vi "Set_Control_Values.vi"(0 "Devices in":T18, 1 "Settings message":T1, 3 "Set Mode":T3, 4 "Timer parameters in":refnum<vi>, 5 "Main Parameters in":T4={"Mode"={"Mode"=enum."Dialog", "Expert?"=FALSE, "Dialog?"=FALSE}, "Stop loop"={"Settings changed?"=FALSE, "Stop?"=refnum}, "Send message"={"Send mode"=enum."Get parameters", "Set parameter list"=0, "Get parameter list"=0, "Reset device"=0, "Length set settings message"=0, "Reset buttons?"=FALSE, "Reset Master?"=enum."General"}, "Write settings"={"Options"=enum."File 1"}, "Settings state"={"MAS locked?"=refnum, "SLV locked?"=refnum}, "Button refs"={"Stop program"=refnum, "Save settings"=refnum, "DAQ mode"=refnum, "Reset settings"=refnum, "Apply settings"=refnum, "Reset MAS"=refnum, "Reset SLV"=refnum, "Local DBase?"=refnum, "Last value DBase"=FALSE, "Database"=refnum, "Calibration"=refnum, "Save settings 2"=refnum}, "Update screen"={"Detector number"=0, "Hardware"=enum."None"}, "Files"={"Path config file"=path "", "Path def. ini file"=path "", "Path ini file 1"=path "", "Path ini file 2"=path "", "Path RBF file"=path ""}, "DB connection"={"connection reference"=refnum, "Connected?"=refnum, "ODBC Name"=""}, "Status_id"=refnum, "Time difference"=refnum, "Satellites"=refnum, "Alignment parameters"=refnum, "Page Statistics 2"=refnum, "Database"=refnum, "Page Statistics"=refnum} {"Update screen"."Detector number" format="%#.0f"; "Send message"."Reset device" format="%x"; "Send message"."Get parameter list" format="%x"; "Send message"."Set parameter list" format="%x"}, 9 "Control Parameters [] in":T19[](array[typedef]) {"Aux Byte Value" format="%02x"; "Max Real Value" format="%#_6e"; "Min Real Value" format="%#_6e"; "dReal/dByte" format="%#_6e"; "Byte Value" format="%02x"; "Identifier" format="%02x"}, 11 "Status/Errors in":refnum<vi>) -> (6 "Main parameters out":T4={"Mode"={"Mode"=enum."Dialog", "Expert?"=FALSE, "Dialog?"=FALSE}, "Stop loop"={"Settings changed?"=FALSE, "Stop?"=refnum}, "Send message"={"Send mode"=enum."Get parameters", "Set parameter list"=0, "Get parameter list"=0, "Reset device"=0, "Length set settings message"=0, "Reset buttons?"=FALSE, "Reset Master?"=enum."General"}, "Write settings"={"Options"=enum."File 1"}, "Settings state"={"MAS locked?"=refnum, "SLV locked?"=refnum}, "Button refs"={"Stop program"=refnum, "Save settings"=refnum, "DAQ mode"=refnum, "Reset settings"=refnum, "Apply settings"=refnum, "Reset MAS"=refnum, "Reset SLV"=refnum, "Local DBase?"=refnum, "Last value DBase"=FALSE, "Database"=refnum, "Calibration"=refnum, "Save settings 2"=refnum}, "Update screen"={"Detector number"=0, "Hardware"=enum."None"}, "Files"={"Path config file"=path "", "Path def. ini file"=path "", "Path ini file 1"=path "", "Path ini file 2"=path "", "Path RBF file"=path ""}, "DB connection"={"connection reference"=refnum, "Connected?"=refnum, "ODBC Name"=""}, "Status_id"=refnum, "Time difference"=refnum, "Satellites"=refnum, "Alignment parameters"=refnum, "Page Statistics 2"=refnum, "Database"=refnum, "Page Statistics"=refnum} {"Update screen"."Detector number" format="%#.0f"; "Send message"."Reset device" format="%x"; "Send message"."Get parameter list" format="%x"; "Send message"."Set parameter list" format="%x"}, 8 "Run twice?":bool, 10 "Control Parameters [] out":T19[](array[typedef]) {"Aux Byte Value" format="%02x"; "Max Real Value" format="%#_6e"; "Min Real Value" format="%#_6e"; "dReal/dByte" format="%#_6e"; "Byte Value" format="%02x"; "Identifier" format="%02x"}, 12 "Slave Settings Message":T1, 14 "Master Settings Message":T1, 15 "Settings ok?":bool)   [LabVIEW 2013]
uses:
  Controls/Control_Parameters.ctl
  Controls/Master.ctl
  Controls/Devices.ctl
  Controls/Main_Parameters.ctl
  Controls/Mode.ctl
  Controls/Stop_Loop.ctl
  Controls/Send_Message.ctl
  Controls/Send_Message_Mode.ctl
  Controls/Write_Settings.ctl
  Controls/Write_Settings_Options.ctl
  Controls/Settings_State.ctl
  Controls/Button_Refs.ctl
  Controls/Update_Screen.ctl
  Controls/Files.ctl
  Controls/DB_Connection.ctl
  database/Connection.llb/Conn ObjectReference.ctl
  Controls/Settings_Message.ctl
  Controls/Setting.ctl
  Controls/Set_Mode.ctl
  Controls/Get_Set_Device_Options.ctl
  Controls/Device_Elements.ctl
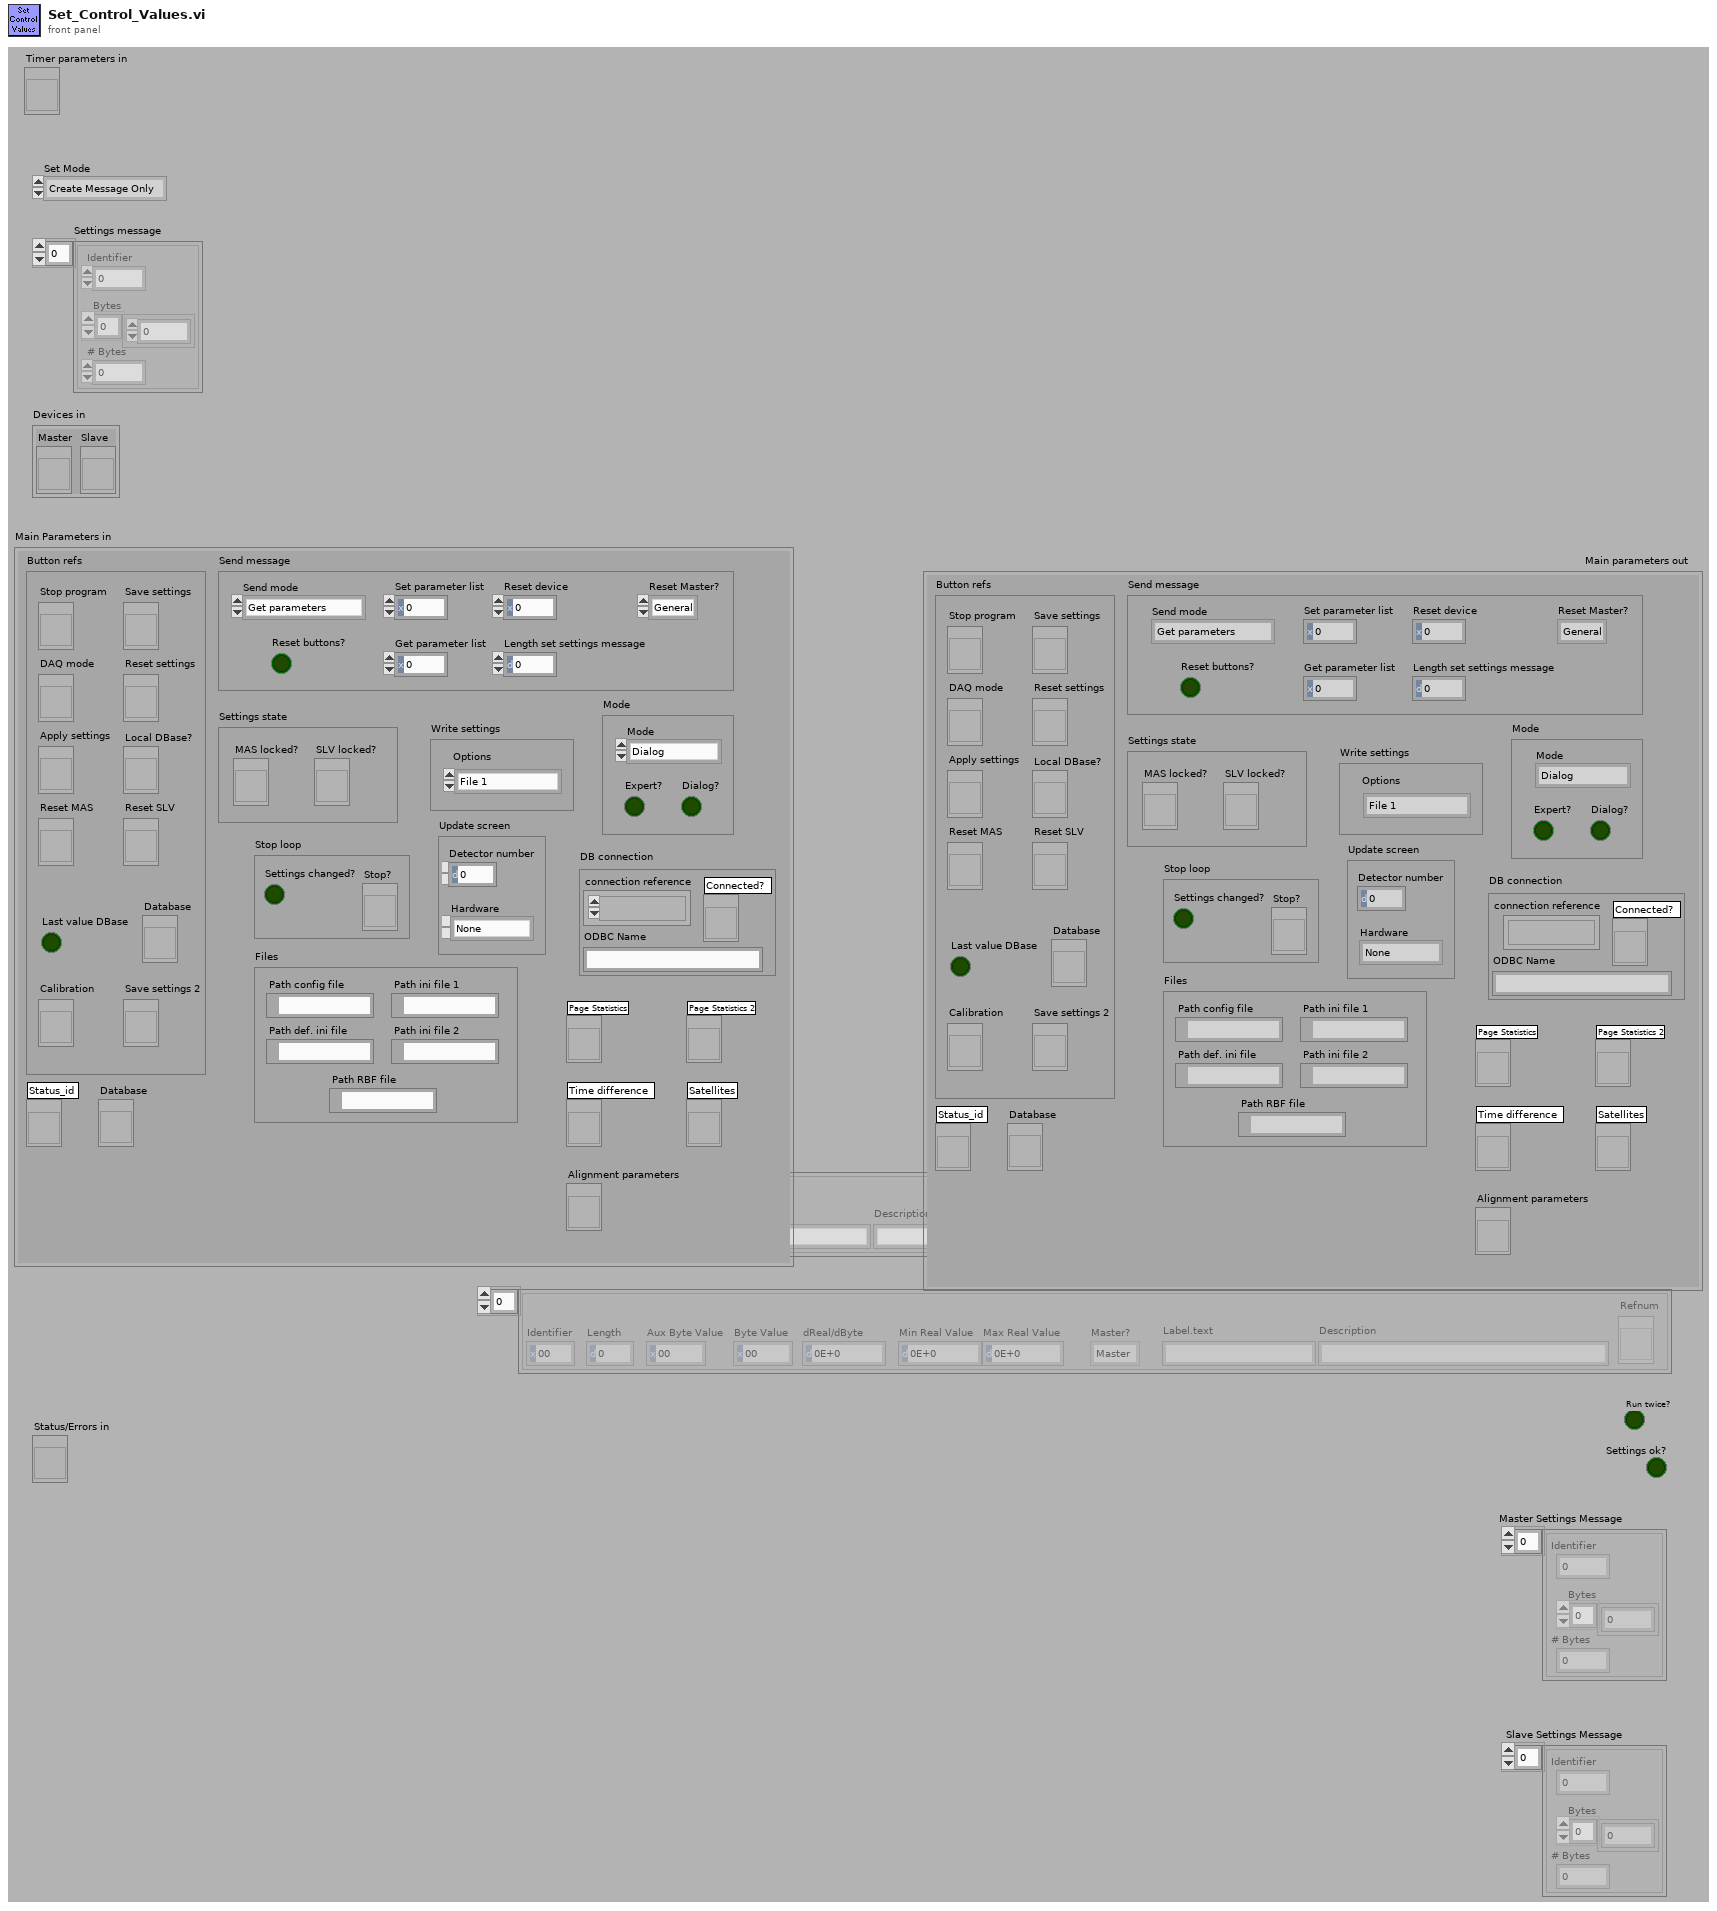
[diagram p1: front panel]
types:
  T1 = typedef "Settings_Message.ctl" = T2[]
  T2 = typedef "Setting.ctl" = cluster{"Identifier":u8, "  Bytes":u8[], "# Bytes":u16}
  T3 = typedef "Set_Mode.ctl" = enum16{"Create Message Only", "Front Panel", "Parameters", "Master", "Slave"}
  T4 = typedef "Main_Parameters.ctl" = cluster{"Mode":T5, "Stop loop":T6, "Send message":T7, "Write settings":T10, "Settings state":T12, "Button refs":T13, "Update screen":T14, "Files":T15, "DB connection":T16, "Status_id":refnum<vi>, "Time difference":refnum<vi>, "Satellites":refnum<vi>, "Alignment parameters":refnum<vi>, "Page Statistics 2":refnum<vi>, "Database":refnum<vi>, "Page Statistics":refnum<vi>}
  T5 = typedef "Mode.ctl" = cluster{"Mode":enum8{"Stop", "Dialog", "Hisparc II", "Hisparc II DAQ", "Alignment"}, "Expert?":bool, "Dialog?":bool}
  T6 = typedef "Stop_Loop.ctl" = cluster{"Settings changed?":bool, "Stop?":refnum<vi>}
  T7 = typedef "Send_Message.ctl" = cluster{"Send mode":T8, "Set parameter list":u8, "Get parameter list":u8, "Reset device":u8, "Length set settings message":i32, "Reset buttons?":bool, "Reset Master?":T9}
  T8 = typedef "Send_Message_Mode.ctl" = enum16{"Get parameters", "Set parameters", "From front panel", "From parameters", "Reset device", "Alignment"}
  T9 = typedef "Master.ctl" = enum16{"Master", "Slave", "General"}
  T10 = typedef "Write_Settings.ctl" = cluster{"Options":T11}
  T11 = typedef "Write_Settings_Options.ctl" = enum16{"File 1", "File 2", "Alignment", "Reset"}
  T12 = typedef "Settings_State.ctl" = cluster{"MAS locked?":refnum<vi>, "SLV locked?":refnum<vi>}
  T13 = typedef "Button_Refs.ctl" = cluster{"Stop program":refnum<vi>, "Save settings":refnum<vi>, "DAQ mode":refnum<vi>, "Reset settings":refnum<vi>, "Apply settings":refnum<vi>, "Reset MAS":refnum<vi>, "Reset SLV":refnum<vi>, "Local DBase?":refnum<vi>, "Last value DBase":bool, "Database":refnum<vi>, "Calibration":refnum<vi>, "Save settings 2":refnum<vi>}
  T14 = typedef "Update_Screen.ctl" = cluster{"Detector number":u16, "Hardware":enum8{"None", "HiSPARC I", "HiSPARC II", "HiSPARC III", "Unknown"}}
  T15 = typedef "Files.ctl" = cluster{"Path config file":path, "Path def. ini file":path, "Path ini file 1":path, "Path ini file 2":path, "Path RBF file":path}
  T16 = typedef "DB_Connection.ctl" = cluster{"connection reference":T17, "Connected?":refnum<vi>, "ODBC Name":string}
  T17 = typedef "Conn ObjectReference.ctl" = refnum<k1>
  T18 = typedef "Devices.ctl" = cluster{"Master":refnum<vi>, "Slave":refnum<vi>}
  T19 = typedef "Control_Parameters.ctl" = cluster{"Identifier":u8, "Length":u16, "Byte Value":u32, "dReal/dByte":dbl, "Min Real Value":dbl, "Max Real Value":dbl, "Master?":T9, "Label.text":string, "Description":string, "Refnum":refnum<vi>, "Aux Byte Value":u32}
  T20 = typedef "Device_Elements.ctl" = enum16{"Default", "Master?", "Connected?", "Status", "Disconnect?", "Handle", "Version number"}
  T21 = typedef "Get_Set_Device_Options.ctl" = enum16{"Get", "Get cluster", "Set"}
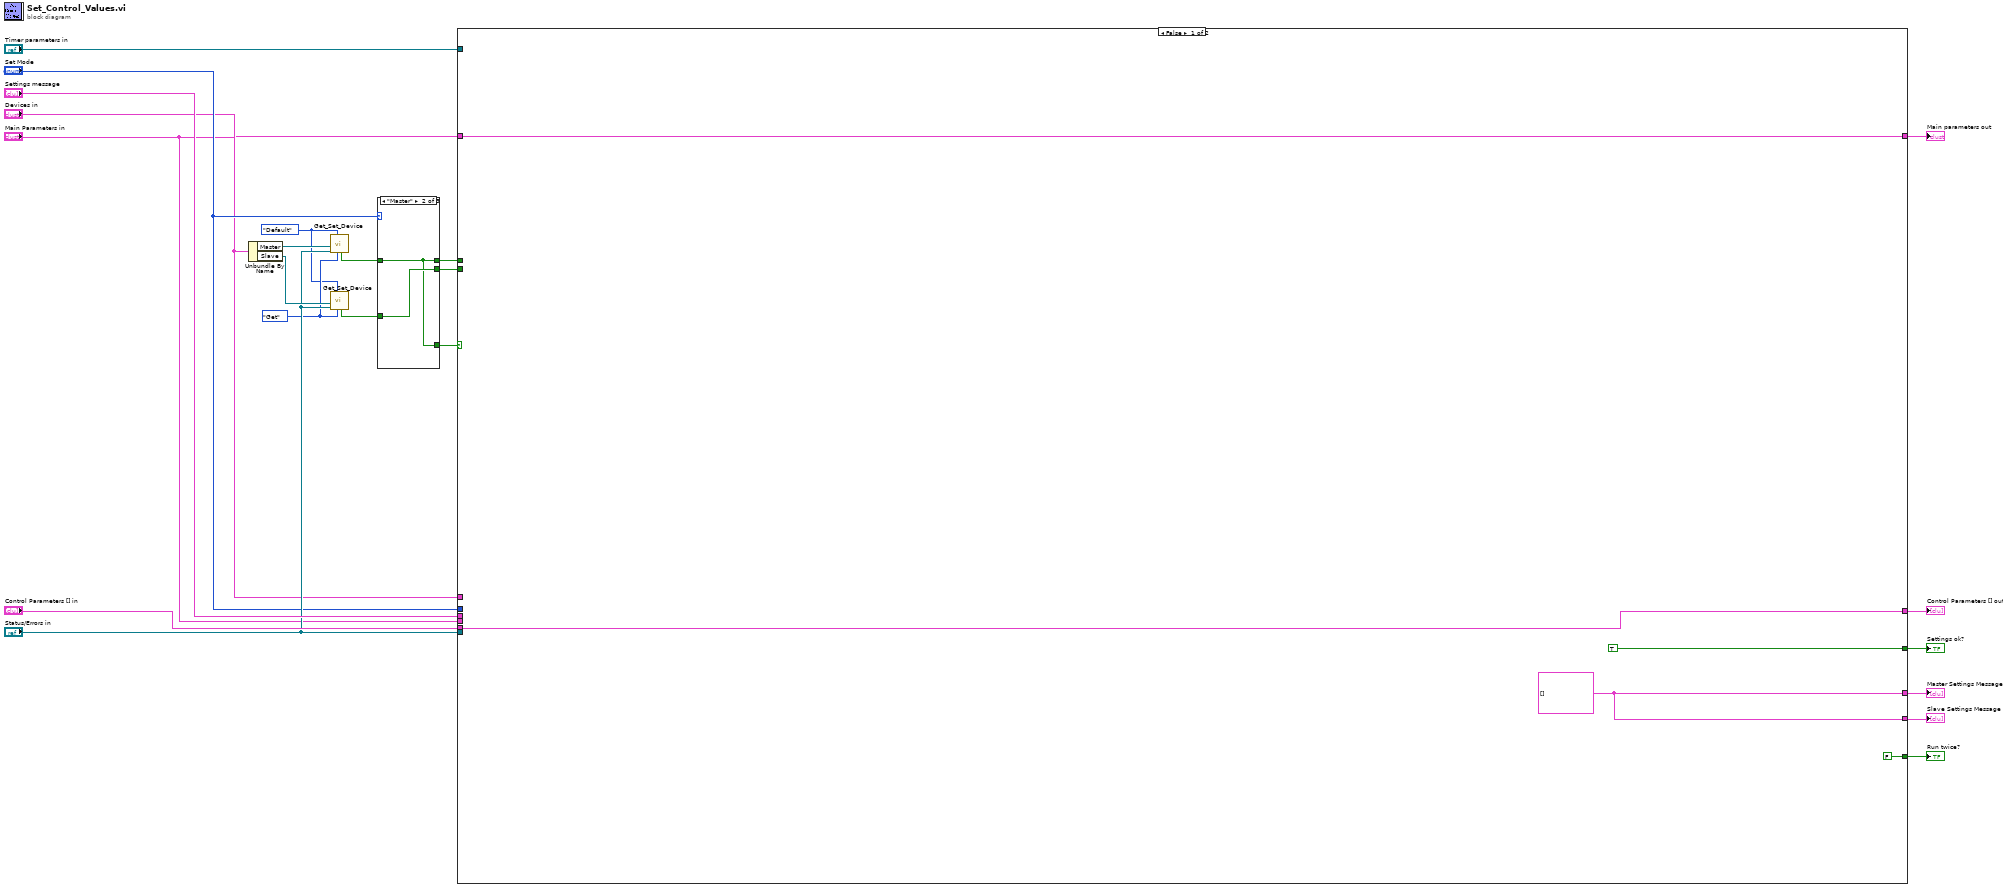
[diagram p0: block diagram]
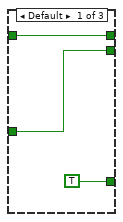
[diagram p2: hidden frame]
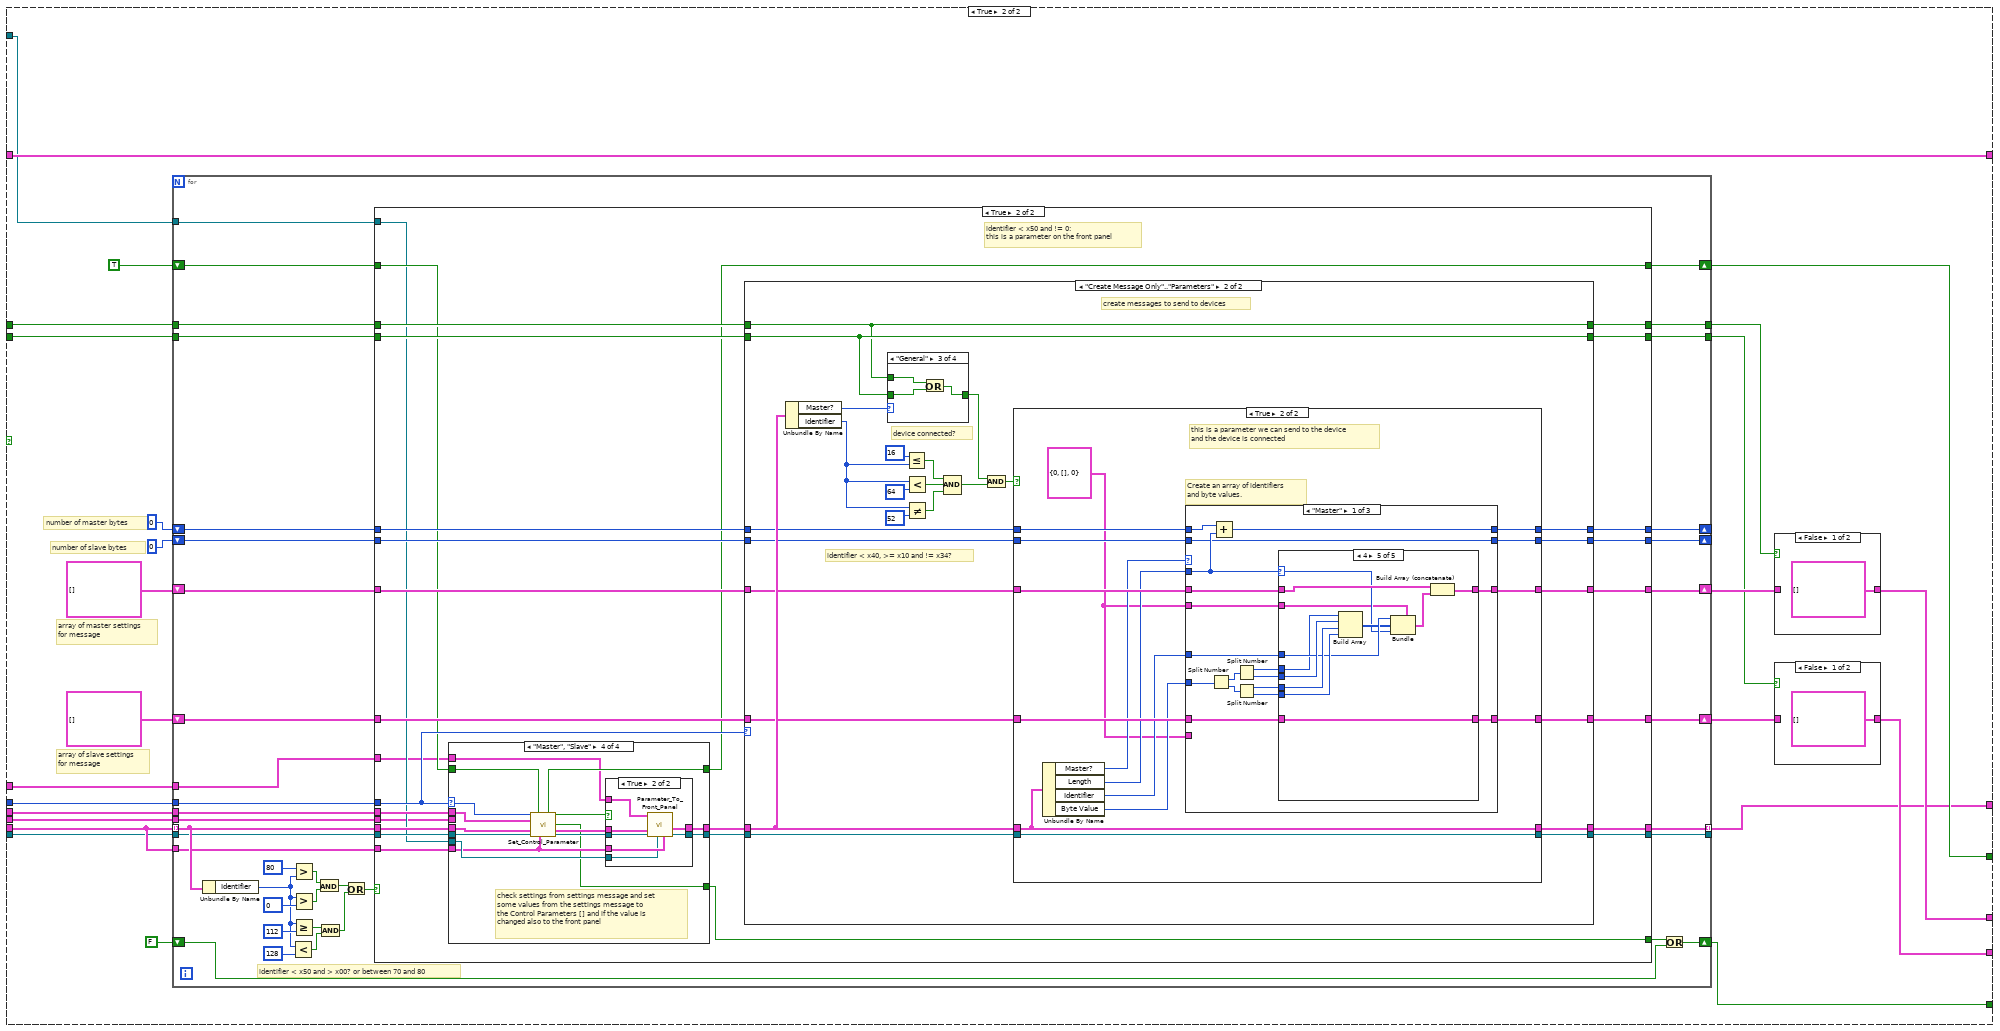
[diagram p4: hidden frame]
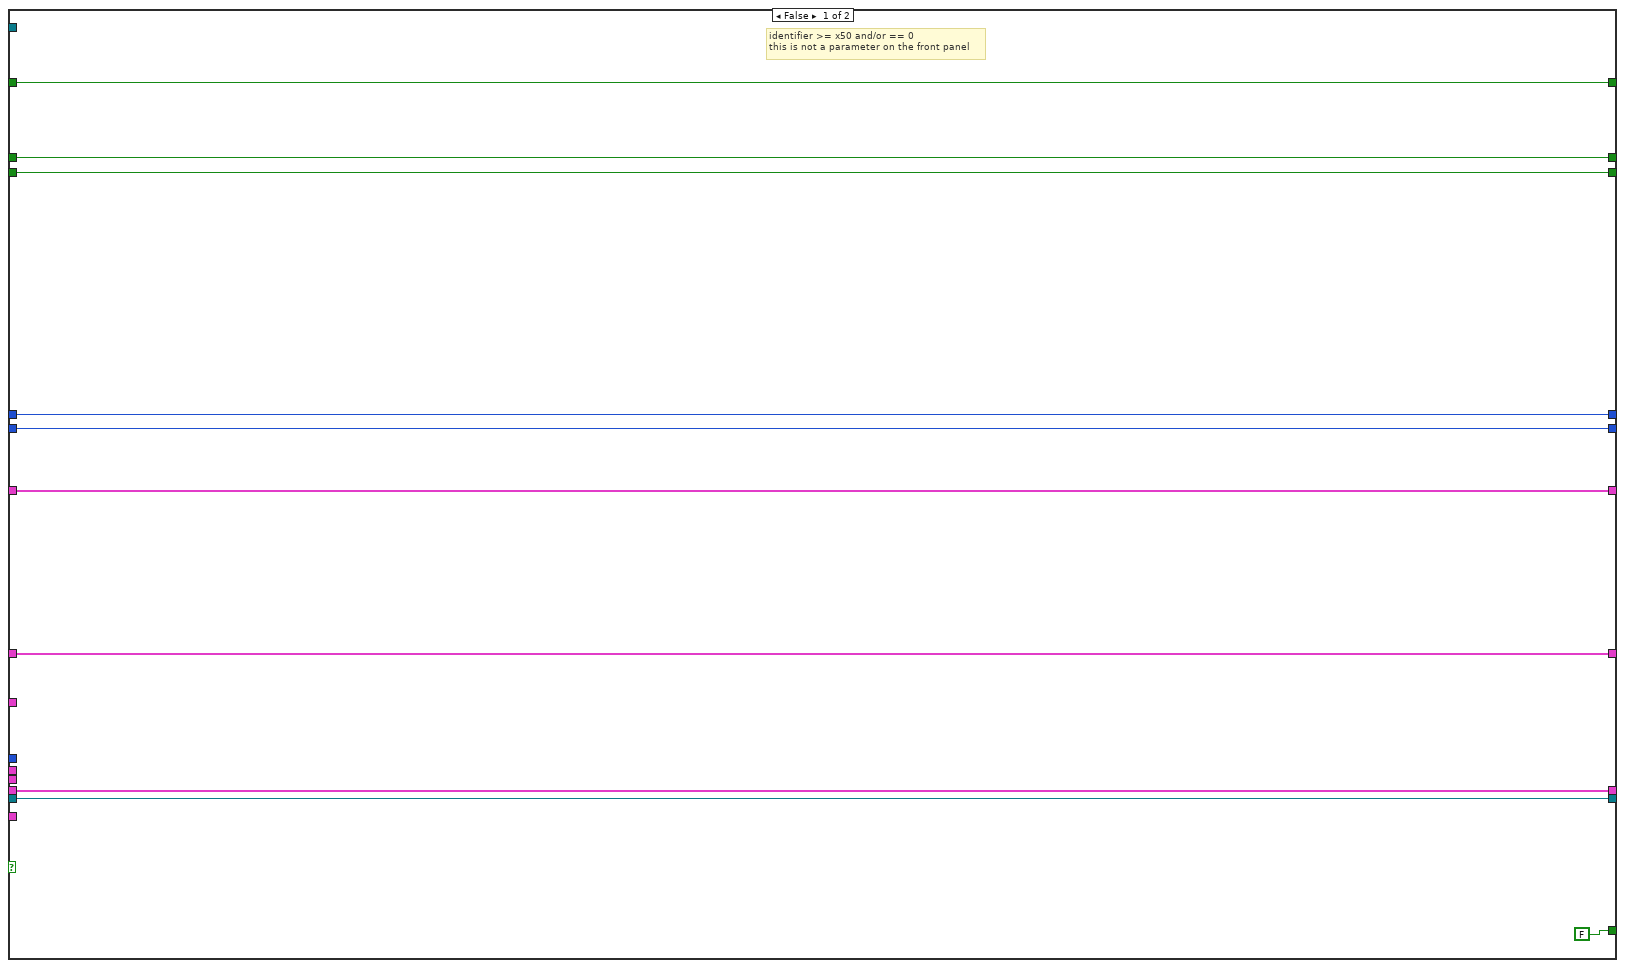
[diagram p7: hidden frame]
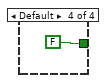
[diagram p11: hidden frame]
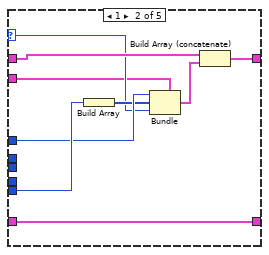
[diagram p14: hidden frame]
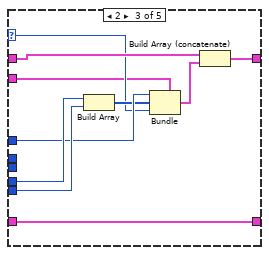
[diagram p15: hidden frame]
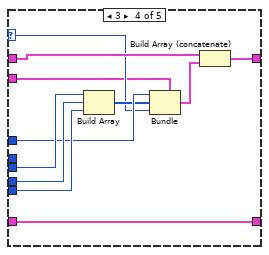
[diagram p16: hidden frame]
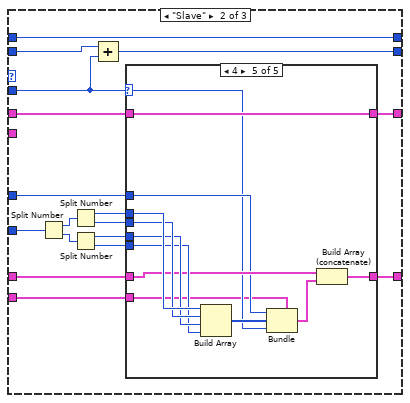
[diagram p17: hidden frame]
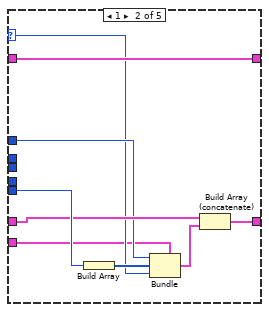
[diagram p19: hidden frame]
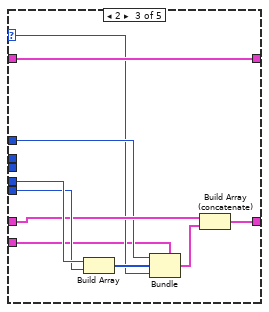
[diagram p20: hidden frame]
diagram:
  w5 = Device_Elements."Default" ("Element")
  w6 = Get_Set_Device_Options."Get" ("Get/Set")
  n1 = Unbundle By Name("Devices in") -> ("Master"=w15:refnum<vi>, "Slave"=w16:refnum<vi>)
  n2 = call "Get_Set_Device.vi"("Get/Set"=w6, "Element"=w5, "Status/Errors in"="Status/Errors in", "Device in"=w15) -> ("Connected?"=w11:bool)  [unwired: 1 in, 6 out]
  n3 = call "Get_Set_Device.vi"("Get/Set"=w6, "Element"=w5, "Status/Errors in"="Status/Errors in", "Device in"=w16) -> ("Connected?"=w10:bool)  [unwired: 1 in, 6 out]
  n4 = case shown="\"Master\"" "Set Mode" {
    tunnel: w11 -> [w25 w26 w29]
    tunnel: w10 -> [w24 w27 w28]
    tunnel: [w25 w26 w29] -> w9
    tunnel: [w24 w27 w28] -> w8
    tunnel: [TRUE w26 w28] -> w7
    frame Default {
    }
    frame "Master" {
    }
    frame "Slave" {
    }
  }
  n5 = case shown="False" w7 {
    tunnel: "Control Parameters [] in" -> [w32 w46]
    tunnel: "Main Parameters in" -> [w33 w59]
    tunnel: [w31 w42] -> w21
    tunnel: [w31 w43] -> w20
    tunnel: [w33 w59] -> w19
    tunnel: [w32 w41] -> w18
    tunnel: "Settings message" -> [_ w48]
    tunnel: w8 -> [_ w37]
    tunnel: w9 -> [_ w38]
    tunnel: "Status/Errors in" -> [_ w45]
    tunnel: [TRUE w44] -> w13
    tunnel: "Set Mode" -> [_ w49]
    tunnel: "Timer parameters in" -> [_ w51]
    tunnel: "Devices in" -> [_ w50]
    tunnel: "Main Parameters in" -> [_ w47]
    tunnel: [FALSE w36] -> w1
    frame False {
      w31 = T1 [] ("Settings message")
    }
    frame True {
      # "array of slave settings\nfor message"
      # "array of master settings\nfor message"
      # "number of slave bytes"
      # "number of master bytes"
      n6 = for {
        tunnel: w46 -> [w102] mode=indexing
        tunnel: w49 -> [w100]
        tunnel: w45 -> [w99]
        tunnel: [w98] -> _
        shift-right: [w96] -> w53
        shift-left: T1 [] ("Settings message") -> [w97]
        shift-right: [w94] -> _
        shift-left: u16 0 -> [w95]
        shift-right: [w92] -> _
        shift-left: u16 0 -> [w93]
        shift-right: [w90] -> w52
        shift-left: T1 [] ("Settings message") -> [w91]
        tunnel: w38 -> [w87]
        tunnel: w37 -> [w86]
        tunnel: [w67] -> w40
        tunnel: [w85] -> w39
        tunnel: w48 -> [w83]
        shift-right: [w81] -> w44
        shift-left: TRUE -> [w82]
        tunnel: w46 -> [w80]
        tunnel: w51 -> [w79]
        tunnel: w50 -> [w78]
        tunnel: w47 -> [w77]
        tunnel: [w66] -> w41 mode=indexing
        shift-right: [w65] -> w36
        shift-left: FALSE -> [w64]
        # "identifier < x50 and > x00? or between 70 and 80"
        n7 = Unbundle By Name(w102) -> ("Identifier"=w71:u8)
        n8 = Less?(x=w71, y=u8 128) -> (x < y?=w70:bool)
        n9 = Greater?(x=u8 80 ("y"), y=w71) -> (0:w89:bool)
        n10 = Greater?(x=w71, y=u8 0) -> (0:w88:bool)
        n11 = Greater Or Equal?(x=w71, y=u8 112) -> (x >= y?=w73:bool)
        n12 = And(x=w89, y=w88) -> (x .and. y?=w75:bool)
        n13 = And(x=w73, y=w70) -> (x .and. y?=w69:bool)
        n14 = Or(x=w75, y=w69) -> (x .or. y?=w74:bool)
        n15 = case shown="True" w74 {
          tunnel: w102 -> [w112 w139]
          tunnel: [w112 w135] -> w66
          tunnel: w100 -> [_ w121]
          tunnel: w99 -> [w111 w138]
          tunnel: [w111 w125] -> w98
          tunnel: w97 -> [w110 w128]
          tunnel: [w110 w134] -> w96
          tunnel: w95 -> [w109 w126]
          tunnel: [w109 w137] -> w94
          tunnel: w93 -> [w108 w127]
          tunnel: [w108 w136] -> w92
          tunnel: w91 -> [w107 w129]
          tunnel: [w107 w133] -> w90
          tunnel: w87 -> [w106 w131]
          tunnel: w86 -> [w105 w130]
          tunnel: [w106 w122] -> w67
          tunnel: [w105 w123] -> w85
          tunnel: w83 -> [_ w120]
          tunnel: w82 -> [w104 w119]
          tunnel: [w104 w118] -> w81
          tunnel: w80 -> [_ w117]
          tunnel: w79 -> [_ w116]
          tunnel: w78 -> [_ w115]
          tunnel: w77 -> [_ w114]
          tunnel: [FALSE ("Run twice?") w113] -> w68
          frame False {
            # "identifier >= x50 and/or == 0\nthis is not a parameter on the front panel"
          }
          frame True {
            # "identifier < x50 and != 0:\nthis is a parameter on the front panel"
            n16 = case shown="\"Master\", \"Slave\"" w121 {
              selector: w121 -> [_ w417 _ w442]
              tunnel: [w404 w414 w434 w449] -> w132
              tunnel: w139 -> [w404 w418 w435 w451]
              tunnel: w138 -> [w403 w419 w437 w452]
              tunnel: [w403 w415 w436 w450] -> w124
              tunnel: w120 -> [_ w407 _ w448]
              tunnel: w119 -> [w402 w411 w433 w447]
              tunnel: [w402 w411 w433 w446] -> w118
              tunnel: w117 -> [_ w408 w432 w439]
              tunnel: w116 -> [_ w410 w431 w445]
              tunnel: w115 -> [_ w409 w430 w444]
              tunnel: w114 -> [_ w406 _ _]
              tunnel: [FALSE ("Run twice?") w405 FALSE ("Run twice?") w438] -> w113
              frame Default {
              }
              frame "Front Panel" {
                # "take value from the front panel\nand copy it to the \"Control Parameters []\""
                n17 = call "Set_Control_Parameter.vi"("Set Mode"=w417, "Settings message"=w407, "Main Parameters in"=w406, "Control Parameter in"=w418, "Status/Errors in"=w419, "Control Parameters [] in"=w408) -> ("Value Changed?"=w412:bool, "Run twice?"=w405:bool, "Control Parameter out"=w413:T19, "Status/Errors out"=w416:refnum<vi>)  [unwired: 2 in, 4 out]
                n18 = case shown="True" w412 {
                  tunnel: w416 -> [w420 w428]
                  tunnel: [w420 w427] -> w415
                  tunnel: [w421 w426] -> w414
                  tunnel: w413 -> [w421 w425]
                  tunnel: w408 -> [_ w424]
                  tunnel: w410 -> [_ w423]
                  tunnel: w409 -> [_ w422]
                  frame False {
                  }
                  frame True {
                    n19 = call "Parameter_To_Front_Panel.vi"("Control Parameters [] in"=w424, "Timer parameters in"=w423, "Status/Errors in"=w428, "Control Parameter in"=w425, "Devices"=w422) -> ("Status/Errors out"=w427:refnum<vi>, "Control Parameter out"=w426:T19)  [unwired: 1 in, 4 out]
                  }
                }
              }
              frame "Parameters" {
                # "take value from the \"Control Parameters []\"\nand copy it to the front panel"
                n20 = call "Parameter_To_Front_Panel.vi"("Control Parameters [] in"=w432, "Timer parameters in"=w431, "Status/Errors in"=w437, "Control Parameter in"=w435, "Devices"=w430) -> ("Status/Errors out"=w436:refnum<vi>, "Control Parameter out"=w434:T19)  [unwired: 1 in, 4 out]
              }
              frame "Master", "Slave" {
                # "check settings from settings message and set\nsome values from the settings message to\nthe Control Parameters [] and if the value is\nchanged also to the front panel"
                n21 = call "Set_Control_Parameter.vi"("Set Mode"=w442, "Settings ok? in"=w447, "Settings message"=w448, "Control Parameter in"=w451, "Status/Errors in"=w452, "Control Parameters [] in"=w439) -> ("Settings ok? out"=w446:bool, "Value Changed?"=w443:bool, "Run twice?"=w438:bool, "Control Parameter out"=w441:T19, "Status/Errors out"=w440:refnum<vi>)  [unwired: 2 in, 3 out]
                n22 = case shown="True" w443 {
                  tunnel: w440 -> [w454 w461]
                  tunnel: [w454 w460] -> w450
                  tunnel: [w453 w459] -> w449
                  tunnel: w439 -> [_ w458]
                  tunnel: w445 -> [_ w457]
                  tunnel: w444 -> [_ w456]
                  tunnel: w441 -> [w453 w455]
                  frame False {
                  }
                  frame True {
                    n23 = call "Parameter_To_Front_Panel.vi"("Control Parameters [] in"=w458, "Timer parameters in"=w457, "Status/Errors in"=w461, "Control Parameter in"=w455, "Devices"=w456) -> ("Status/Errors out"=w460:refnum<vi>, "Control Parameter out"=w459:T19)  [unwired: 1 in, 4 out]
                  }
                }
              }
            }
            n24 = case shown="\"Create Message Only\"..\"Parameters\"" w121 {
              tunnel: [w147 w168] -> w137
              tunnel: [w146 w167] -> w136
              tunnel: [w143 w166] -> w135
              tunnel: [w145 w165] -> w134
              tunnel: [w144 w164] -> w133
              tunnel: w132 -> [w143 w163]
              tunnel: w131 -> [w141 w155]
              tunnel: w130 -> [w140 w156]
              tunnel: w129 -> [w144 w162]
              tunnel: w128 -> [w145 w161]
              tunnel: w127 -> [w146 w160]
              tunnel: w126 -> [w147 w159]
              tunnel: [w142 w158] -> w125
              tunnel: w124 -> [w142 w157]
              tunnel: [w140 w156] -> w123
              tunnel: [w141 w155] -> w122
              frame Default {
                # "don't create messages to send to devices\n('Master' and 'Slave' cases: here we only check settings from settings message)"
              }
              frame "Create Message Only".."Parameters" {
                # "create messages to send to devices"
                # "device connected?"
                # "identifier < x40, >= x10 and != x34?"
                n25 = Unbundle By Name(w163) -> ("Master?"=w169:T9, "Identifier"=w150:u8)
                n26 = case shown="\"General\"" w169 {
                  tunnel: w155 -> [w173 _ w176 _]
                  tunnel: w156 -> [_ w174 w175 _]
                  tunnel: [w173 w174 w177 FALSE ("Connected?")] -> w170
                  frame "Master" {
                  }
                  frame "Slave" {
                  }
                  frame "General" {
                    n27 = Or(x=w176, y=w175) -> (x .or. y?=w177:bool)
                  }
                  frame Default {
                  }
                }
                n28 = Less Or Equal?(x=u8 16, y=w150) -> (x <= y?=w152:bool)
                n29 = Less?(x=w150, y=u8 64) -> (x < y?=w151:bool)
                n30 = Not Equal?(x=w150, y=u8 52) -> (x != y?=w148:bool)
                n31 = Compound Arithmetic op=AND(w152, w151, w148) -> (w153:bool)
                n32 = And(x=w170, y=w153) -> (x .and. y?=w171:bool)
                n33 = case shown="True" w171 {
                  tunnel: [w184 w197] -> w166
                  tunnel: w163 -> [w184 w197]
                  tunnel: w161 -> [w181 w199]
                  tunnel: [w181 w198] -> w165
                  tunnel: w159 -> [w183 w191]
                  tunnel: w160 -> [w182 w190]
                  tunnel: [w183 w196] -> w168
                  tunnel: [w182 w195] -> w167
                  tunnel: w162 -> [w180 w194]
                  tunnel: [w180 w193] -> w164
                  tunnel: [w179 w187] -> w158
                  tunnel: w157 -> [w179 w187]
                  frame False {
                    # "this is not a parameter we can send to the device\nand/or the device is not connected"
                  }
                  frame True {
                    w185 = T2 {"Identifier"=0, "  Bytes"=[], "# Bytes"=0} ("Setting")
                    # "this is a parameter we can send to the device\nand the device is connected"
                    # "Create an array of identifiers\nand byte values."
                    n34 = Unbundle By Name(w197) -> ("Master?"=w186:T9, "Length"=w189:u16, "Identifier"=w188:u8, "Byte Value"=w192:u32)
                    n35 = case shown="\"Master\"" w186 {
                      tunnel: w189 -> [w202 w263 w324]
                      tunnel: w192 -> [w214 w275 w338]
                      tunnel: w188 -> [w209 w270 w333]
                      tunnel: w199 -> [w208 w269 w332]
                      tunnel: [w207 w268 w331] -> w198
                      tunnel: w191 -> [w206 w262 w330]
                      tunnel: [w205 w262 w329] -> w196
                      tunnel: w190 -> [w201 w265 w326]
                      tunnel: [w201 w264 w325] -> w195
                      tunnel: w194 -> [w204 w267 w328]
                      tunnel: [w203 w266 w327] -> w193
                      tunnel: w185 -> [w200 _ w323]
                      tunnel: w185 -> [_ w261 w322]
                      frame "Master" {
                        n36 = Split Number(x=w214) -> (hi(x)=w215:u16, lo(x)=w216:u16)
                        n37 = Add(x=w206, y=w202) -> (x+y=w205:u16)
                        n38 = Split Number(x=w215) -> (hi(x)=w210:u8, lo(x)=w211:u8)
                        n39 = Split Number(x=w216) -> (hi(x)=w212:u8, lo(x)=w213:u8)
                        n40 = case shown="4" w202 {
                          selector: w202 -> [_ w220 w229 w239 w251]
                          tunnel: w213 -> [_ w227 w236 w246 w258]
                          tunnel: w212 -> [_ _ w237 w247 w259]
                          tunnel: w211 -> [_ _ _ w248 w260]
                          tunnel: w210 -> [_ _ _ _ w250]
                          tunnel: [w218 w225 w234 w244 w256] -> w207
                          tunnel: w209 -> [_ w223 w232 w242 w254]
                          tunnel: w208 -> [w218 w224 w233 w243 w255]
                          tunnel: w204 -> [w217 w221 w230 w240 w252]
                          tunnel: [w217 w221 w230 w240 w252] -> w203
                          tunnel: w200 -> [_ w219 w228 w238 w249]
                          frame Default {
                          }
                          frame 1 {
                            n41 = Build Array(w227) -> (w222:u8[])
                            n42 = Bundle(cluster=w219, "Identifier"=w223, "Bytes"=w222, "# Bytes"=w220) -> (w226:T2)
                            n43 = Build Array (concatenate)(w224, w226) -> (w225:T1)
                          }
                          frame 2 {
                            n44 = Build Array(w237, w236) -> (w231:u8[])
                            n45 = Bundle(cluster=w228, "Identifier"=w232, "Bytes"=w231, "# Bytes"=w229) -> (w235:T2)
                            n46 = Build Array (concatenate)(w233, w235) -> (w234:T1)
                          }
                          frame 3 {
                            n47 = Build Array(w248, w247, w246) -> (w241:u8[])
                            n48 = Bundle(cluster=w238, "Identifier"=w242, "Bytes"=w241, "# Bytes"=w239) -> (w245:T2)
                            n49 = Build Array (concatenate)(w243, w245) -> (w244:T1)
                          }
                          frame 4 {
                            n50 = Build Array(w250, w260, w259, w258) -> (w253:u8[])
                            n51 = Bundle(cluster=w249, "Identifier"=w254, "Bytes"=w253, "# Bytes"=w251) -> (w257:T2)
                            n52 = Build Array (concatenate)(w255, w257) -> (w256:T1)
                          }
                        }
                      }
                      frame "Slave" {
                        n53 = Split Number(x=w275) -> (hi(x)=w276:u16, lo(x)=w277:u16)
                        n54 = Split Number(x=w276) -> (hi(x)=w271:u8, lo(x)=w272:u8)
                        n55 = Split Number(x=w277) -> (hi(x)=w273:u8, lo(x)=w274:u8)
                        n56 = Add(x=w265, y=w263) -> (x+y=w264:u16)
                        n57 = case shown="4" w263 {
                          selector: w263 -> [_ w281 w290 w300 w311]
                          tunnel: w274 -> [_ w288 w297 w307 w318]
                          tunnel: w273 -> [_ _ w298 w308 w319]
                          tunnel: w272 -> [_ _ _ w309 w320]
                          tunnel: w271 -> [_ _ _ _ w321]
                          tunnel: [w279 w282 w291 w301 w312] -> w268
                          tunnel: w270 -> [_ w283 w292 w302 w313]
                          tunnel: w269 -> [w279 w282 w291 w301 w312]
                          tunnel: w267 -> [w278 w286 w295 w305 w316]
                          tunnel: [w278 w287 w296 w306 w317] -> w266
                          tunnel: w261 -> [_ w280 w289 w299 w310]
                          frame Default {
                          }
                          frame 1 {
                            n58 = Build Array(w288) -> (w285:u8[])
                            n59 = Bundle(cluster=w280, "Identifier"=w283, "Bytes"=w285, "# Bytes"=w281) -> (w284:T2)
                            n60 = Build Array (concatenate)(w286, w284) -> (w287:T1)
                          }
                          frame 2 {
                            n61 = Build Array(w298, w297) -> (w294:u8[])
                            n62 = Bundle(cluster=w289, "Identifier"=w292, "Bytes"=w294, "# Bytes"=w290) -> (w293:T2)
                            n63 = Build Array (concatenate)(w295, w293) -> (w296:T1)
                          }
                          frame 3 {
                            n64 = Build Array(w309, w308, w307) -> (w304:u8[])
                            n65 = Bundle(cluster=w299, "Identifier"=w302, "Bytes"=w304, "# Bytes"=w300) -> (w303:T2)
                            n66 = Build Array (concatenate)(w305, w303) -> (w306:T1)
                          }
                          frame 4 {
                            n67 = Build Array(w321, w320, w319, w318) -> (w315:u8[])
                            n68 = Bundle(cluster=w310, "Identifier"=w313, "Bytes"=w315, "# Bytes"=w311) -> (w314:T2)
                            n69 = Build Array (concatenate)(w316, w314) -> (w317:T1)
                          }
                        }
                      }
                      frame "General" {
                        n70 = Split Number(x=w338) -> (hi(x)=w339:u16, lo(x)=w340:u16)
                        n71 = Add(x=w330, y=w324) -> (x+y=w329:u16)
                        n72 = Split Number(x=w339) -> (hi(x)=w334:u8, lo(x)=w335:u8)
                        n73 = Split Number(x=w340) -> (hi(x)=w336:u8, lo(x)=w337:u8)
                        n74 = Add(x=w326, y=w324) -> (x+y=w325:u16)
                        n75 = case shown="1" w324 {
                          selector: w324 -> [_ w345 w358 w372 w389]
                          tunnel: w337 -> [_ w355 w368 w382 w397]
                          tunnel: w336 -> [_ _ w369 w383 w398]
                          tunnel: w335 -> [_ _ _ w384 w399]
                          tunnel: w334 -> [_ _ _ _ w400]
                          tunnel: [w342 w349 w362 w376 w392] -> w331
                          tunnel: w333 -> [_ w347 w360 w374 w388]
                          tunnel: w332 -> [w342 w348 w361 w375 w391]
                          tunnel: w328 -> [w341 w353 w366 w380 w395]
                          tunnel: [w341 w354 w367 w381 w396] -> w327
                          tunnel: w323 -> [_ w344 w357 w370 w386]
                          tunnel: w322 -> [_ w343 w356 w371 w385]
                          frame Default {
                          }
                          frame 1 {
                            n76 = Build Array(w355) -> (w346:u8[])
                            n77 = Build Array(w355) -> (w352:u8[])
                            n78 = Bundle(cluster=w344, "Identifier"=w347, "Bytes"=w346, "# Bytes"=w345) -> (w350:T2)
                            n79 = Bundle(cluster=w343, "Identifier"=w347, "Bytes"=w352, "# Bytes"=w345) -> (w351:T2)
                            n80 = Build Array (concatenate)(w348, w350) -> (w349:T1)
                            n81 = Build Array (concatenate)(w353, w351) -> (w354:T1)
                          }
                          frame 2 {
                            n82 = Build Array(w369, w368) -> (w359:u8[])
                            n83 = Build Array(w369, w368) -> (w365:u8[])
                            n84 = Bundle(cluster=w357, "Identifier"=w360, "Bytes"=w359, "# Bytes"=w358) -> (w363:T2)
                            n85 = Bundle(cluster=w356, "Identifier"=w360, "Bytes"=w365, "# Bytes"=w358) -> (w364:T2)
                            n86 = Build Array (concatenate)(w361, w363) -> (w362:T1)
                            n87 = Build Array (concatenate)(w366, w364) -> (w367:T1)
                          }
                          frame 3 {
                            n88 = Build Array(w384, w383, w382) -> (w373:u8[])
                            n89 = Build Array(w384, w383, w382) -> (w379:u8[])
                            n90 = Bundle(cluster=w370, "Identifier"=w374, "Bytes"=w373, "# Bytes"=w372) -> (w377:T2)
                            n91 = Bundle(cluster=w371, "Identifier"=w374, "Bytes"=w379, "# Bytes"=w372) -> (w378:T2)
                            n92 = Build Array (concatenate)(w375, w377) -> (w376:T1)
                            n93 = Build Array (concatenate)(w380, w378) -> (w381:T1)
                          }
                          frame 4 {
                            n94 = Build Array(w400, w399, w398, w397) -> (w390:u8[])
                            n95 = Build Array(w400, w399, w398, w397) -> (w394:u8[])
                            n96 = Bundle(cluster=w386, "Identifier"=w388, "Bytes"=w390, "# Bytes"=w389) -> (w387:T2)
                            n97 = Bundle(cluster=w385, "Identifier"=w388, "Bytes"=w394, "# Bytes"=w389) -> (w393:T2)
                            n98 = Build Array (concatenate)(w391, w387) -> (w392:T1)
                            n99 = Build Array (concatenate)(w395, w393) -> (w396:T1)
                          }
                        }
                      }
                    }
                  }
                }
              }
            }
          }
        }
        n100 = Or(x=w68, y=w64) -> (x .or. y?=w65:bool)
      }
      n101 = case shown="False" w40 {
        tunnel: [T1 [] ("Master Settings Message") w63] -> w43
        tunnel: w53 -> [_ w63]
        frame False {
        }
        frame True {
        }
      }
      n102 = case shown="False" w39 {
        tunnel: [T1 [] ("Master Settings Message") w61] -> w42
        tunnel: w52 -> [_ w61]
        frame False {
        }
        frame True {
        }
      }
    }
  }
  "Control Parameters [] out" <- w18
  "Main parameters out" <- w19
  "Slave Settings Message" <- w21
  "Master Settings Message" <- w20
  "Settings ok?" <- w13
  "Run twice?" <- w1
